vi "Extract SV URLs.vi"(8 "error in (no error)":errorcluster, 10 "Page":string, 11 "Device Reference in":T1 format="%.0x") -> (0 "error out":errorcluster, 1 "SV":T2, 2 "Channel Refs":T1[](array[typedef]) format="%.0x", 3 "Device Reference out":T1=18446744073709551615 format="%.0x")   [LabVIEW 2017, in "Shared Variables CD 2.0 Engine.lvlib"]
uses:
  Shared Variables CD 2.0 Engine.lvlib
  <vilib>/NI Veristand/Custom Device API/Custom Device Item Ref.ctl
  Shared DataTypes/URLs.ctl
  <vilib>/Utility/error.llb/Error Cluster From Error Code.vi
  Shared/SV Global.vi
  <vilib>/ErrorRing/Error Ring.xnode
  <vilib>/NI Veristand/Custom Device API/Custom Device API.lvlib
  <vilib>/NI Veristand/Custom Device Tools/Custom Device Utility Library/Custom Device Utility Library.lvlib
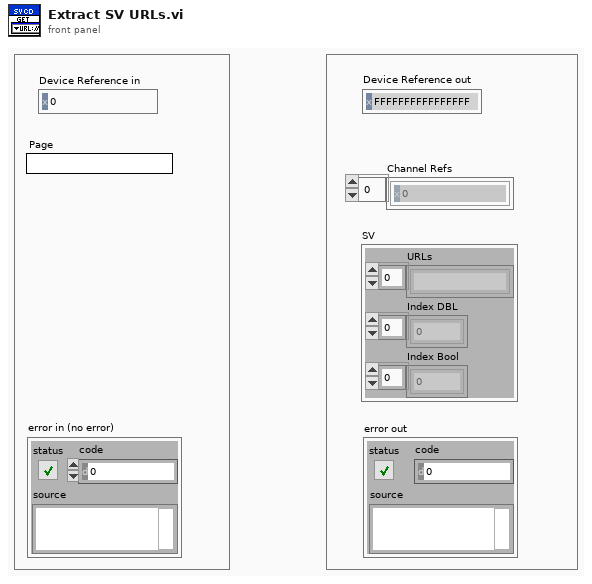
[diagram p1: front panel]
types:
  T1 = typedef "Custom Device API.lvlib/Custom Device Item Ref.ctl" = u64
  T2 = typedef "URLs.ctl" = cluster{"URLs":string[], "Index DBL":i32[], "Index Bool":i32[]}
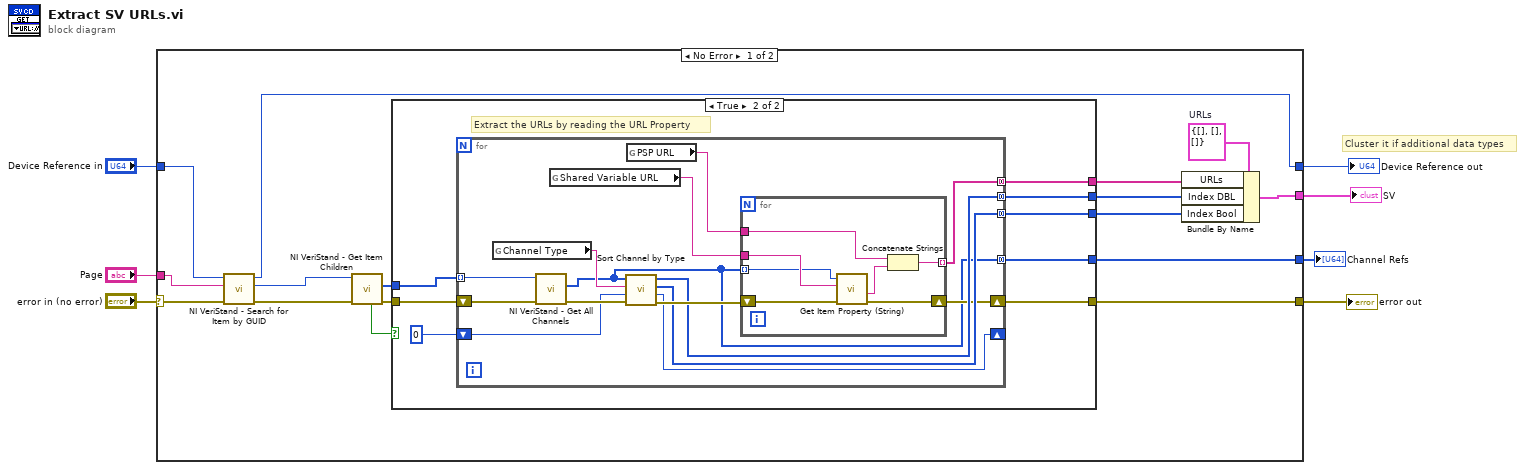
[diagram p0: block diagram]
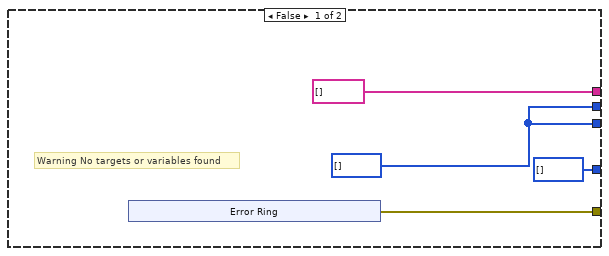
[diagram p2: hidden frame]
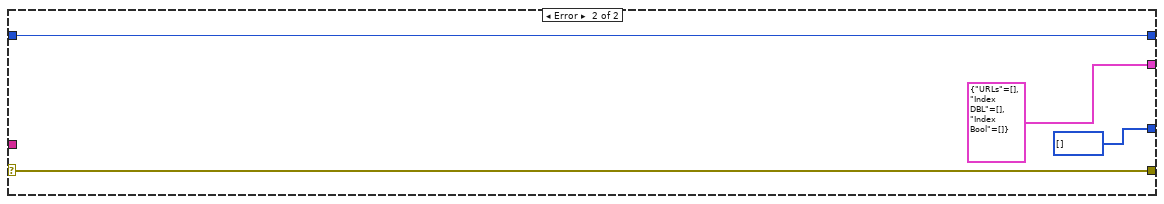
[diagram p3: hidden frame]
diagram:
  # "Cluster it if additional data types"
  n1 = case shown="No Error" "error in (no error)" {
    selector: "error in (no error)" -> [w14 w64]
    tunnel: [w23 w64] -> w7
    tunnel: "Device Reference in" -> [w22 w65]
    tunnel: "Page" -> [w16 _]
    tunnel: [w15 w65] -> w4
    tunnel: [w11 T2 {"URLs"=[], "Index DBL"=[], "Index Bool"=[]} ("URLs")] -> w2
    tunnel: [w8 T1[] [] ("Channel Refs")] -> w1
    frame No Error {
      w13 = T2 {"URLs"=[], "Index DBL"=[], "Index Bool"=[]}  # URLs
      n2 = call <vilib>:"NI VeriStand - Search for Item by GUID.vi"("error in"=w14, "Item GUID"=w16, "Section Ref in"=w22) -> ("error out"=w21:errorcluster, "Item Ref"=w17:T1, "Section Ref out"=w15:T1)  [unwired: 5 in, 1 out]
      n3 = call <vilib>:"NI VeriStand - Get Item Children.vi"("error in (no error)"=w21, "Item Ref in"=w17) -> ("error out"=w20:errorcluster, "Child Refs"=w18:T1[], "Found"=w19:bool)  [unwired: 6 in, 1 out]
      n4 = case shown="True" w19 {
        tunnel: w18 -> [_ w40]
        tunnel: w20 -> [_ w39]
        tunnel: [w27 w38] -> w23
        tunnel: [string[] [] w37] -> w12
        tunnel: [w25 w36] -> w10
        tunnel: [w25 w35] -> w9
        tunnel: [T1[] [] ("Channel Refs") w33] -> w8
        frame False {
          w25 = i32[] [] ("Index DBL")
          # "Warning No targets or variables found"
          n5 = xnode "Error Ring"() -> ("error out"=w27:errorcluster)
        }
        frame True {
          # "Extract the URLs by reading the URL Property"
          n6 = for {
            tunnel: w40 -> [w54] mode=indexing
            shift-right: [w44] -> w38
            shift-left: w39 -> [w53]
            tunnel: [w47] -> w37 mode=concatenating
            tunnel: [w46] -> w36 mode=concatenating
            tunnel: [w45] -> w35 mode=concatenating
            shift-right: [w42] -> _
            shift-left: 0 -> [w43]
            tunnel: [w41] -> w33 mode=concatenating
            n7 = global read "SV Global.vi" "Channel Type"() -> (w52:string)
            n8 = call <vilib>:"NI VeriStand - Get All Channels.vi"("error in"=w53, "Section Ref in"=w54) -> ("error out"=w51:errorcluster, "Channel Refs"=w41:T1[])  [unwired: 6 in, 2 out]
            n9 = global read "SV Global.vi" "Shared Variable URL"() -> (w48:string)
            n10 = call "Sort Channel by Type.vi"("error in (no error)"=w51, "Index"=w43, "Property"=w52, "Specified Channel Ref List"=w41) -> ("error out"=w50:errorcluster, "Last Index"=w42:i32, "Index Bool"=w45:i32[], "Index DBL"=w46:i32[])  [unwired: 4 in]
            n11 = global read "SV Global.vi" "PSP URL"() -> (w49:string)
            n12 = for {
              tunnel: w49 -> [w58]
              shift-right: [w60] -> w44
              shift-left: w50 -> [w61]
              tunnel: w48 -> [w59]
              tunnel: [w57] -> w47 mode=indexing
              tunnel: w41 -> [w55] mode=indexing
              n13 = call <vilib>:"Get Item Property (String).vi"("error in (no error)"=w61, "Property Name"=w59, "Item Ref in"=w55) -> ("error out"=w60:errorcluster, "Value"=w56:string)  [unwired: 5 in, 2 out]
              n14 = Concatenate Strings(w58, w56) -> (w57:string)
            }
          }
        }
      }
      n15 = Bundle By Name(cluster=w13, "URLs"=w12, "Index DBL"=w10, "Index Bool"=w9) -> (w11:T2)
    }
    frame Error {
    }
  }
  "error out" <- w7
  "Device Reference out" <- w4
  "SV" <- w2
  "Channel Refs" <- w1
